vi "fwEndComms.vi"(0 "fw cluster":cluster{"FW Handle":u32, "init?":i16}) -> ()   [LabVIEW 2015]
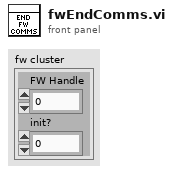
[diagram p1: front panel]
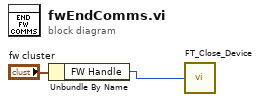
[diagram p0: block diagram]
diagram:
  n1 = Unbundle By Name("fw cluster") -> ("FW Handle"=w2:u32)
  n2 = call "FT_Close_Device.vi"("Handle"=w2) -> ()  [unwired: 1 out]
